vi "extract required data channels.vi"(8 "Cluster in":T1={"rigChannels"=[], "rigUnits"=[], "logging"=FALSE, "chartRef"=refnum, "dataTableRef"=refnum, "channelCount"=0, "trendIndex"=0, "channels"={"massflow"=0, "PR"=0, "recircTemp"=0}, "History"={"speedlines"=[], "liveTail"={"mDot"=[], "pRatio"=[]}, "current"={"mDot"=0.0, "pRatio"=0.0}, "insertPoint"=0, "tempHistory"=[]}, "filter"=FALSE, "filterLength"=0, "tableUpdate"=0, "limitValues"=[[0.0, 45000.0], [0.0, 100.0], [0.0, 100.0], [10.0, 100.0], [0.0, 100.0], [10.0, 35.0], [0.0, 100.0], [0.0, 100.0], [99000.0, 300000.0], [-5000.0, 5000.0], [99000.0, 300000.0], [-0.01, 0.3], [-0.01, 4.5], [-0.1, 100.0], [1.0, 8.0], [1.0, 5.0], [0.0, 100.0], [0.0, 100.0], [0.0, 100.0], [-100.0, 45000.0], [-0.1, 1.0], [0.8, 2.0], [90000.0, 110000.0], [15.0, 35.0], [0.0, 0.0], [0.0, 0.0], [0.0, 0.0], [0.0, 0.0]]}, 11 "averagedData":dbl[](array[numeric])) -> (0 "cluster out":T1={"rigChannels"=[], "rigUnits"=[], "logging"=FALSE, "chartRef"=refnum, "dataTableRef"=refnum, "channelCount"=0, "trendIndex"=0, "channels"={"massflow"=0, "PR"=0, "recircTemp"=0}, "History"={"speedlines"=[], "liveTail"={"mDot"=[], "pRatio"=[]}, "current"={"mDot"=0.0, "pRatio"=0.0}, "insertPoint"=0, "tempHistory"=[]}, "filter"=FALSE, "filterLength"=0, "tableUpdate"=0, "limitValues"=[[0.0, 45000.0], [0.0, 100.0], [0.0, 100.0], [10.0, 100.0], [0.0, 100.0], [10.0, 35.0], [0.0, 100.0], [0.0, 100.0], [99000.0, 300000.0], [-5000.0, 5000.0], [99000.0, 300000.0], [-0.01, 0.3], [-0.01, 4.5], [-0.1, 100.0], [1.0, 8.0], [1.0, 5.0], [0.0, 100.0], [0.0, 100.0], [0.0, 100.0], [-100.0, 45000.0], [-0.1, 1.0], [0.8, 2.0], [90000.0, 110000.0], [15.0, 35.0], [0.0, 0.0], [0.0, 0.0], [0.0, 0.0], [0.0, 0.0]]}, 1 "temp history":dbl[][](array[numeric]), 2 "recircT":dbl)   [LabVIEW 2018]
uses:
  custom sub vis/speedlineData.ctl
  <vilib>/Analysis/baseanly.llb/Mean (DBL).vi
  <vilib>/Analysis/NI_AALBase.lvlib
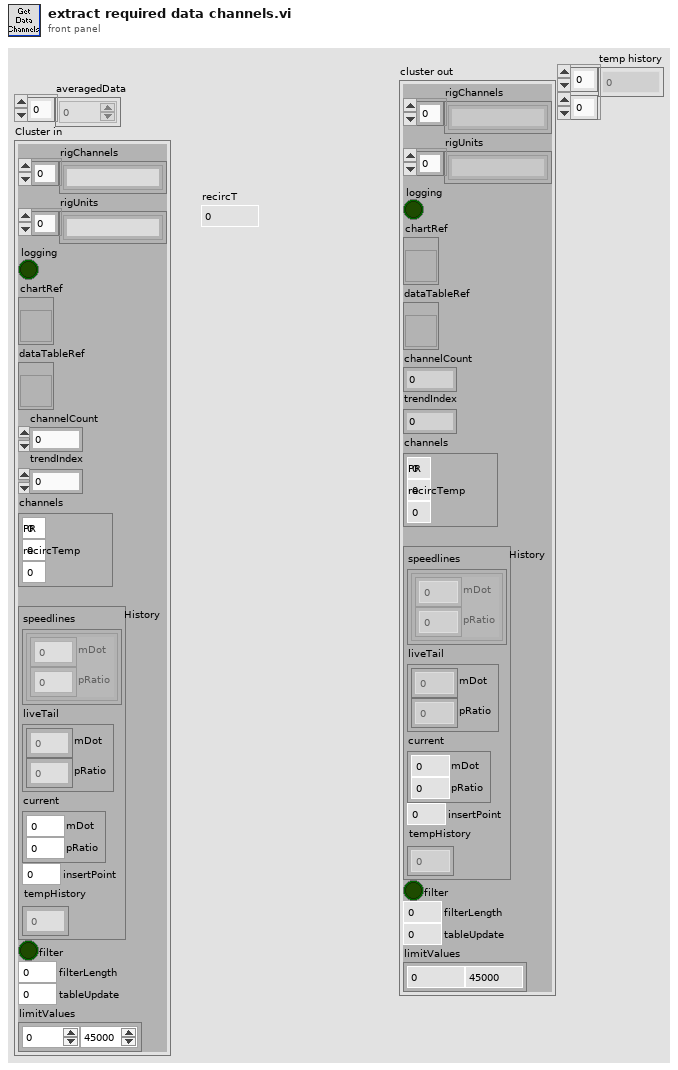
[diagram p1: front panel]
types:
  T1 = typedef "speedlineData.ctl" = cluster{"rigChannels":string[], "rigUnits":string[], "logging":bool, "chartRef":refnum<vi>, "dataTableRef":refnum<vi>, "channelCount":i32, "trendIndex":i32, "channels":cluster{"massflow":i32, "PR":i32, "recircTemp":i32}, "History":cluster{"speedlines":cluster{"mDot":dbl[], "pRatio":dbl[]}[], "liveTail":cluster{"mDot":dbl[], "pRatio":dbl[]}, "current":cluster{"mDot":dbl, "pRatio":dbl}, "insertPoint":i32, "tempHistory":dbl[][]}, "filter":bool, "filterLength":i32, "tableUpdate":i16, "limitValues":dbl[][]}
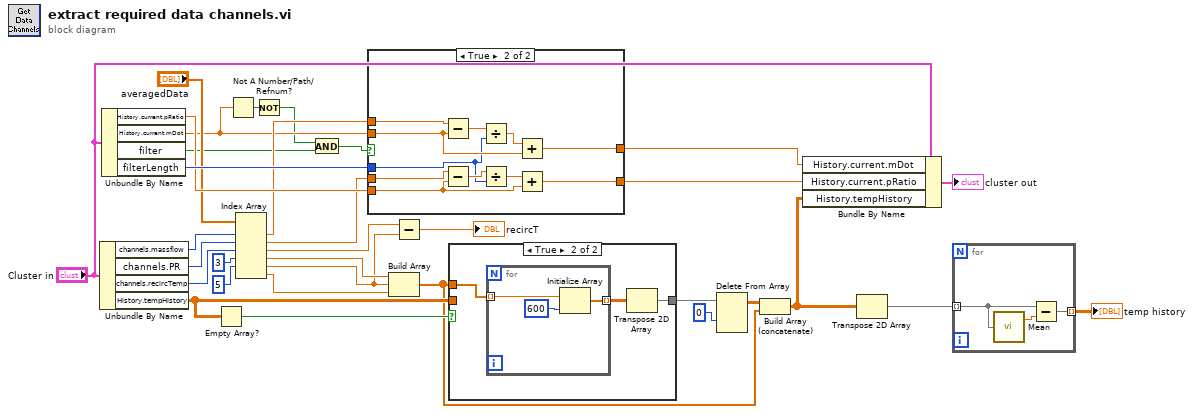
[diagram p0: block diagram]
diagram:
  n1 = Unbundle By Name("Cluster in") -> ("channels.massflow"=w26:i32, "channels.PR"=w25:i32, "channels.recircTemp"=w24:i32, "History.tempHistory"=w10:dbl[][])
  n2 = Unbundle By Name("Cluster in") -> ("History.current.pRatio"=w32:dbl, "History.current.mDot"=w5:dbl, "filter"=w4:bool, "filterLength"=w33:i32)
  n3 = Empty Array?(array=w10) -> (empty?=w11:bool)
  n4 = Not A Number/Path/Refnum?(number/path/refnum=w5) -> (NaN/Path/Refnum?=w3:bool)
  n5 = Index Array(array="averagedData", index #1=w26, index #2=w25, index #3=w24, index #4=3 ("index"), index #5=5 ("index")) -> (element #1=w21:dbl, element #2=w22:dbl, element #3=w23:dbl, element #4=w18:dbl, element #5=w6:dbl, element #6=w17:dbl)  [unwired: 1 in]
  n6 = Not(x=w3) -> (.not. x?=w2:bool)
  n7 = And(x=w2, y=w4) -> (x .and. y?=w1:bool)
  n8 = case shown="True" w1 {
    tunnel: w32 -> [_ w44]
    tunnel: w33 -> [_ w39]
    tunnel: [w34 w43] -> w27
    tunnel: w5 -> [_ w40]
    tunnel: [w35 w38] -> w28
    tunnel: w22 -> [w34 w37]
    tunnel: w21 -> [w35 w36]
    frame False {
    }
    frame True {
      n9 = Subtract(x=w36, y=w40) -> (x-y=w41:dbl)
      n10 = Subtract(x=w37, y=w44) -> (x-y=w46:dbl)
      n11 = Divide(x=w41, y=w39) -> (x/y=w42:dbl)
      n12 = Divide(x=w46, y=w39) -> (x/y=w45:dbl)
      n13 = Add(x=w42, y=w40) -> (x+y=w38:dbl)
      n14 = Add(x=w45, y=w44) -> (x+y=w43:dbl)
    }
  }
  n15 = Build Array(w18, w6, w17) -> (w9:dbl[])
  n16 = Subtract(x=w23, y=w6) -> (x-y=→"recircT":dbl)
  n17 = case shown="True" w11 {
    tunnel: w10 -> [w47 _]
    tunnel: w9 -> [_ w50]
    tunnel: [w47 w48] -> w8
    frame False {
    }
    frame True {
      n18 = for {
        tunnel: w50 -> [w52] mode=indexing
        tunnel: [w51] -> w49 mode=indexing
        n19 = Initialize Array(w52, 600 ("dimension size")) -> (w51:dbl[])
      }
      n20 = Transpose 2D Array(2D array=w49) -> (transposed array=w48:dbl[][])
    }
  }
  n21 = Delete From Array(array=w8, index (row)=0) -> (array with subset deleted=w16:dbl[][])  [unwired: 2 in, 1 out]
  n22 = Build Array (concatenate)(w16, w9) -> (w14:dbl[][])
  n23 = Bundle By Name(cluster="Cluster in", "History.current.mDot"=w28, "History.current.pRatio"=w27, "History.tempHistory"=w14) -> (→"cluster out":T1)
  n24 = Transpose 2D Array(2D array=w14) -> (transposed array=w13:dbl[][])
  n25 = for {
    tunnel: w13 -> [w55] mode=indexing
    tunnel: [w54] -> w12 mode=indexing
    n26 = call-poly <vilib>:"Mean.vi"("X"=w55) -> ("mean"=w56:dbl)  [unwired: 1 out]
    n27 = Subtract(x=w55, y=w56) -> (x-y=w54:dbl[])
  }
  "temp history" <- w12
